vi "measurement.vi"() -> ()   [LabVIEW 2026]
uses:
  <vilib>/Distrio/LabbitMQ/Connection/Connection.lvclass
  <vilib>/Distrio/LabbitMQ/Channel/exchange_type_enum.ctl
  <vilib>/Distrio/LabbitMQ/Connection/connection_parameters_cluster.ctl
  <vilib>/Distrio/LabbitMQ/Channel/exchange_declare_cluster.ctl
  <vilib>/Distrio/LabbitMQ/Queue/Queue.lvclass
  <vilib>/Distrio/LabbitMQ/Channel/Channel.lvclass
panel:
  out "error out":errorcluster
  out "Waveform Graph":dbl[](graph)
  in  "Stop":bool
  out "consumer: received message":string
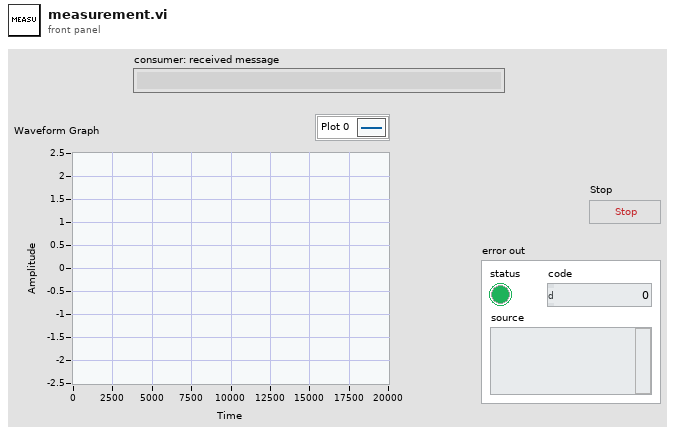
[diagram p1: front panel]
types:
  T1 = typedef "Channel.lvclass/exchange_declare_cluster.ctl" = cluster{"durable (F)":bool, "autoDelete (F)":bool, "561934e089]], mscorlib, Version=0.0.0.0, Culture=neutral, PublicKeyToken=b77a5c561934e089\targuments":refnum<k24>}
  T2 = typedef "Connection.lvclass/connection_parameters_cluster.ctl" = cluster{"host name":string, "port":i32, "user name":string, "password":string, "virtual host":string}
  T3 = typedef "Channel.lvclass/exchange_type_enum.ctl" = enum16{"direct", "topic", "fanout", "headers"}
  T4 = cluster{"sampling_rate_hz":dbl, "duration_s":dbl, "fault_enabled":bool, "correlation_id":string}
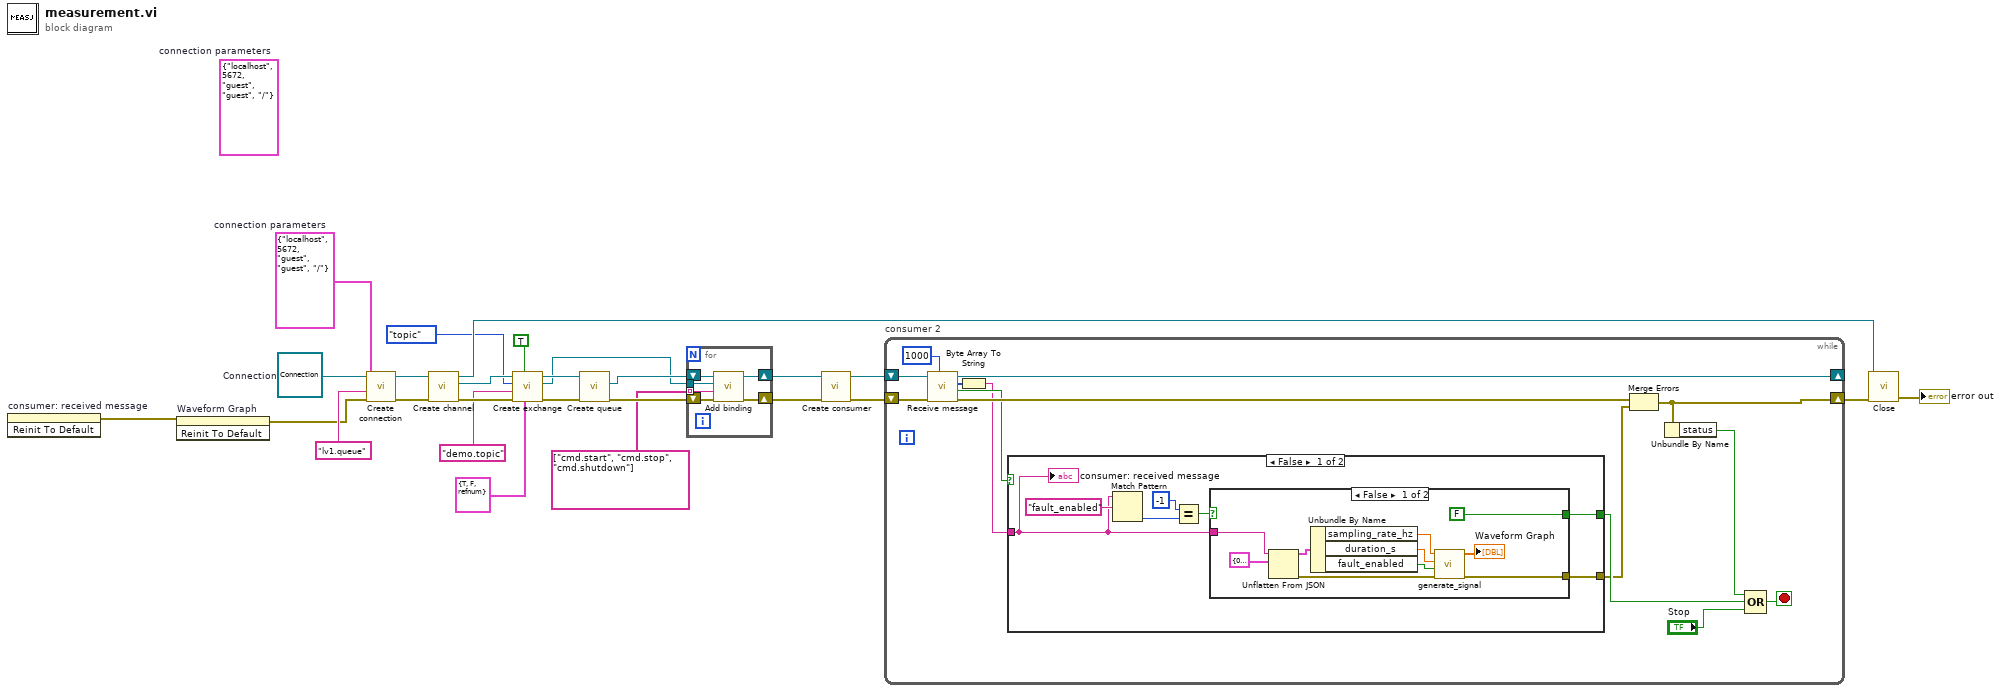
[diagram p0: block diagram]
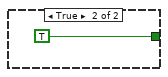
[diagram p2: hidden frame]
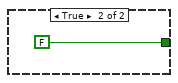
[diagram p3: hidden frame]
diagram:
  w6 = T2 {"host name"="localhost", "port"=5672, "user name"="guest", "password"="guest", "virtual host"="/"}  # connection parameters
  (unwired) T2 {"host name"="localhost", "port"=5672, "user name"="guest", "password"="guest", "virtual host"="/"}  # connection parameters
  w26 = refnum<class "Connection.lvclass"> refnum  # Connection
  n1 = invoke on="consumer: received message" class="Str" method="Reinit To Default"() -> (error out=w2:errorcluster)  [unwired: 3 in, 2 out]
  n2 = invoke on="Waveform Graph" class="WFGraph (strict)" method="Reinit To Default"(error in=w2) -> (error out=w3:errorcluster)  [unwired: 2 in, 2 out]
  n3 = call <vilib>:"Create connection.vi"("error in (no error)"=w3, "ID"="lv1.queue", "connection parameters"=w6, "Connection in"=w26) -> ("error out"=w24:errorcluster, "Connection out"=w25:refnum<class "Connection.lvclass">)  [unwired: 6 in]
  n4 = call <vilib>:"Create channel.vi"("error in (no error)"=w24, "Connection in"=w25) -> ("error out"=w21:errorcluster, "channel"=w20:refnum<class "Channel.lvclass">, "Connection out"=w22:refnum<class "Connection.lvclass">)  [unwired: 7 in]
  n5 = call <vilib>:"Create exchange.vi"("ExchangeDeclare properties"=T1 {"durable (F)"=TRUE, "autoDelete (F)"=FALSE, "561934e089]], mscorlib, Version=0.0.0.0, Culture=neutral, PublicKeyToken=b77a5c561934e089\targuments"=refnum}, "use ExchangeDeclare properties? (F)"=TRUE, "error in (no error)"=w21, "exchange name"="demo.topic", "exchange type"=exchange_type_enum."topic", "Channel in"=w20) -> ("error out"=w15:errorcluster, "Exchange.lvclass"=w13:refnum<class "Exchange.lvclass">, "Channel out"=w14:refnum<class "Channel.lvclass">)  [unwired: 3 in]
  n6 = call <vilib>:"Create queue.vi"("error in (no error)"=w15, "Channel in"=w14) -> ("error out"=w18:errorcluster, "Queue.lvclass"=w16:refnum<class "Queue.lvclass">)  [unwired: 7 in, 1 out]
  n7 = for {
    tunnel: w13 -> [w29]
    tunnel: string[] ["cmd.start", "cmd.stop", "cmd.shutdown"] ("routing key") -> [w28] mode=indexing
    shift-right: [w27] -> w10
    shift-left: w18 -> [w32]
    shift-right: [w31] -> w17
    shift-left: w16 -> [w30]
    n8 = call <vilib>:"Add binding.vi"("error in (no error)"=w32, "binding key"=w28, "Exchange.lvclass"=w29, "Consumer in"=w30) -> ("error out"=w27:errorcluster, "Consumer out"=w31:refnum<class "Queue.lvclass">)  [unwired: 6 in]
  }
  n9 = call <vilib>:"Create consumer.vi"("error in (no error)"=w10, "Queue in"=w17) -> ("error out"=w9:errorcluster, "Queue out"=w12:refnum<class "Queue.lvclass">)  [unwired: 8 in]
  n10 = while "consumer 2" {
    shift-right: [w33] -> w23
    shift-left: w9 -> [w45]
    shift-right: [w40] -> _
    shift-left: w12 -> [w44]
    stop <- w41 stop-if-true
    n11 = call <vilib>:"Receive message.vi"("millisecondsTimeout"=1000, "error in (no error)"=w45, "Consumer in"=w44) -> ("error out"=w43:errorcluster, "timed out?"=w37:bool, "message body"=w46:u8[], "Consumer out"=w40:refnum<class "Queue.lvclass">)  [unwired: 3 in, 2 out]
    n12 = Byte Array To String(unsigned byte array=w46) -> (string=w35:string)
    n13 = case shown="False" w37 {
      tunnel: [w50 FALSE] -> w36
      tunnel: w35 -> [w47 _]
      tunnel: [w48 _] -> w34
      frame False {
        n14 = Match Pattern(string=w47, regular expression="fault_enabled") -> (offset past match=w52:i32)  [unwired: 1 in, 3 out]
        n15 = Equal?(x=-1, y=w52) -> (x = y?=w49:bool)
        n16 = case shown="False" w49 {
          tunnel: [FALSE TRUE] -> w50
          tunnel: w47 -> [w63 _]
          tunnel: [w60 _] -> w48
          frame False {
            n17 = Unflatten From JSON(JSON string=w63, type and defaults=T4 {"sampling_rate_hz"=0.0, "duration_s"=0.0, "fault_enabled"=FALSE, "correlation_id"=""}) -> (value=w58:T4, error out=w61:errorcluster)  [unwired: 5 in]
            n18 = Unbundle By Name(w58) -> ("sampling_rate_hz"=w57:dbl, "duration_s"=w56:dbl, "fault_enabled"=w55:bool)
            n19 = call "generate_signal.vi"("error in (no error)"=w61, "fault_enabled"=w55, "duration_s"=w56, "sampling_rate_hz"=w57) -> ("error out"=w60:errorcluster, "measured values"=→"Waveform Graph":dbl[])  [unwired: 6 in]
          }
          frame True {
          }
        }
        "consumer: received message" <- w47
      }
      frame True {
      }
    }
    n20 = Merge Errors(w43, w34) -> (w33:errorcluster)
    n21 = Unbundle By Name(w33) -> ("status"=w42:bool)
    n22 = Compound Arithmetic op=OR(w42, w36, "Stop") -> (w41:bool)
  }
  n23 = call <vilib>:"Close.vi"("error in (no error)"=w23, "Connection in"=w22) -> ("error out"=→"error out":errorcluster)  [unwired: 8 in, 1 out]
